vi "Init.vi"(8 "error in (no error)":errorcluster) -> (0 "error out":errorcluster, 3 "App out":refnum<class "App.lvclass">)   [LabVIEW 2022 SP3, in "VMR-Deck.lvlib" / "App.lvclass"]
uses:
  App.lvclass
  App.lvclass/App.ctl
  VMR/VMR.lvclass
  WebServer/WebServer.lvclass
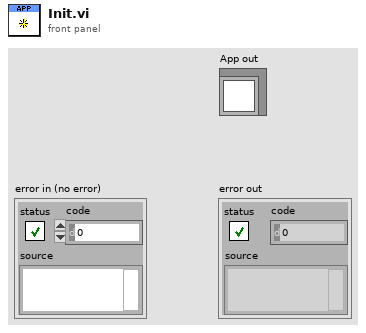
[diagram p1: front panel]
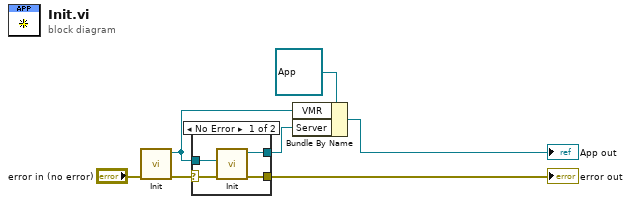
[diagram p0: block diagram]
diagram:
  n1 = call "Init.vi"("error in (no error)"="error in (no error)") -> ("error out"=w5:errorcluster, "VMR out"=w1:refnum<class "VMR.lvclass">)  [unwired: 9 in]
  n2 = case shown="No Error" w5 {
    selector: w5 -> [w11 w12]
    tunnel: [w10 w12] -> w4
    tunnel: [w9 _] -> w2
    tunnel: w1 -> [w8 _]
    frame No Error {
      n3 = call "Init.vi"("error in (no error)"=w11, "VMR"=w8) -> ("error out"=w10:errorcluster, "WebServer out"=w9:refnum<class "WebServer.lvclass">)  [unwired: 8 in]
    }
    frame Error {
    }
  }
  "error out" <- w4
  n4 = Bundle By Name(cluster=refnum<class "App.lvclass"> refnum ("App in"), "VMR"=w1, "Server"=w2) -> (→"App out":refnum<class "App.lvclass">)
